vi "read_data_linear_loadX_mt_connect_R(SubVI).vi"(11 "URL":string="http://amrcadp:5000/current?&path=//") -> ()   [LabVIEW 2017]
uses:
  <vilib>/regexp/Match Regular Expression.xnode
  <vilib>/addons/internet/NI_InternetTK_Core_VIs.lvlib
panel:
  out "trimmed string":string
  out "concatenated string 3":string
  out "content 4":string
  out "empty? 2":bool
  out "content1 2":string
  out "concatenated string 2":string
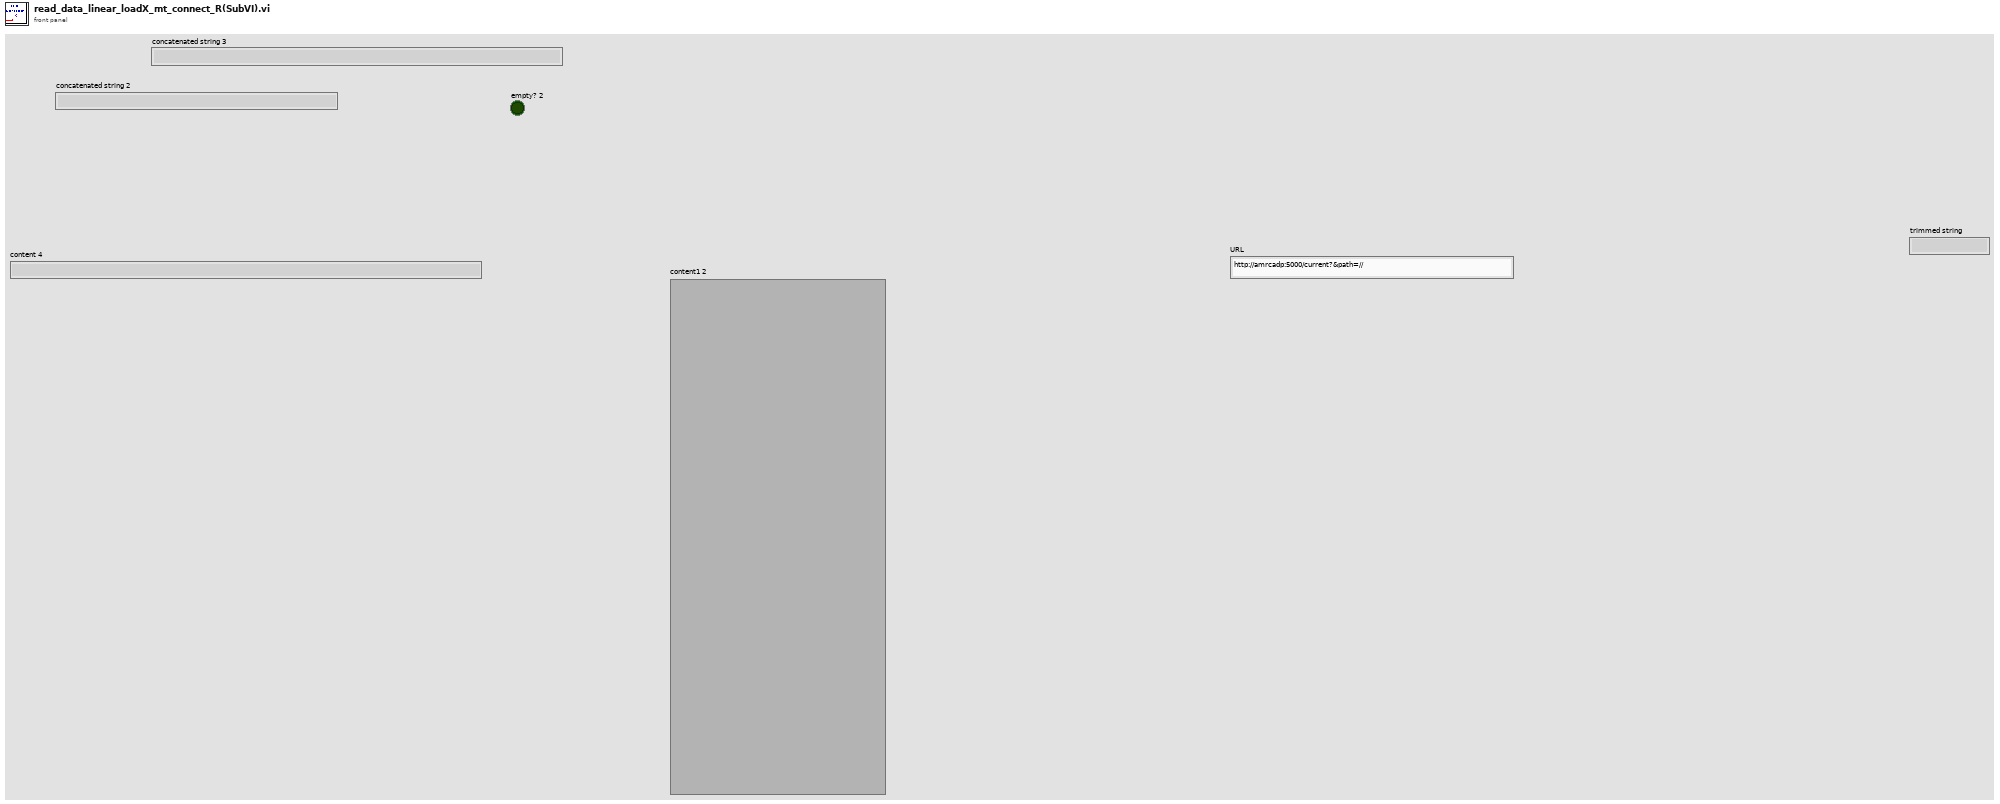
[diagram p1: front panel]
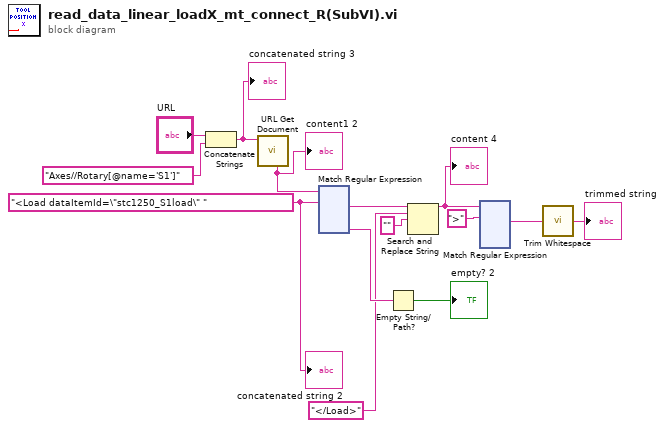
[diagram p0: block diagram]
diagram:
  w3 = "<Load dataItemId=\"stc1250_S1load\" " ("regular expression")
  n1 = Concatenate Strings("URL", "Axes//Rotary[@name='S1']" ("string")) -> (w8:string)
  "concatenated string 3" <- w8
  n2 = call <vilib>:"URL Get Document.vi"("URL"=w8) -> ("content"=w11:string)  [unwired: 6 in, 4 out]
  "content1 2" <- w11
  n3 = xnode "Match Regular Expression"("input string"=w11, "regular expression"=w3) -> ("after match"=w12:string, "submatch 1"=w9:string)  [unwired: 4 in, 4 out]
  n4 = Empty String/Path?(string/path=w9) -> (empty?=→"empty? 2":bool)
  n5 = Search and Replace String(input string=w12, search string="</Load>" ("string"), replace string="" ("string")) -> (result string=w13:string)  [unwired: 5 in, 3 out]
  "content 4" <- w13
  n6 = xnode "Match Regular Expression"("input string"=w13, "regular expression"=">" ("string")) -> ("after match"=w14:string)  [unwired: 4 in, 5 out]
  n7 = call <vilib>:"Trim Whitespace.vi"("string"=w14) -> ("trimmed string"=→"trimmed string":string)  [unwired: 1 in]
  "concatenated string 2" <- w3
